vi "TCP-IP Link._Test_Node2.vi"() -> ()   [LabVIEW 2024, in "EQMF.lvlib" / "TCP-IP.lvlib"]
uses:
  TCP-IP.lvlib
  Controls/TCP-IP Link.Config.ctl
  Controls/TCP-IP Link.Status.ctl
  Queues/Q.Element.ctl
  Controls/TCP-IP Link.Options.ctl
  Controls/TCP-IP Link.Packet Format.ctl
  Queues/Queue Utils.lvlib
panel:
  in  "Options":T1={"Status Notify En"=TRUE, "Auto Connect"=TRUE, "Packet Format"=enum."First 2 Bytes is Length (U16)"}
  in  "Clear Error":bool
  in  "Name":string="Node2"
  out "Error Out":errorcluster
  out "Status Active":bool
  in  "Get Status":bool
  in  "Set Config":bool
  in  "Disconnect":bool
  in  "Connect":bool
  in  "Status":T3={"Cmd"="Task", "Sub"="TCP-IP Status", "Data1"=variant, "Data2"=variant}
  in  "Rcv Data":T3={"Cmd"="Task", "Sub"="TCP-IP Rcv", "Data1"=variant, "Data2"=variant}
  out "Status":T4
  in  "Config":T5={"IP"="127.0.0.1", "Port"=8510, "Listener"=FALSE}
  out "Connected":bool
  in  "Exit":bool
  out "Rcv Data":string
  in  "Send Data":string
  in  "Send":bool
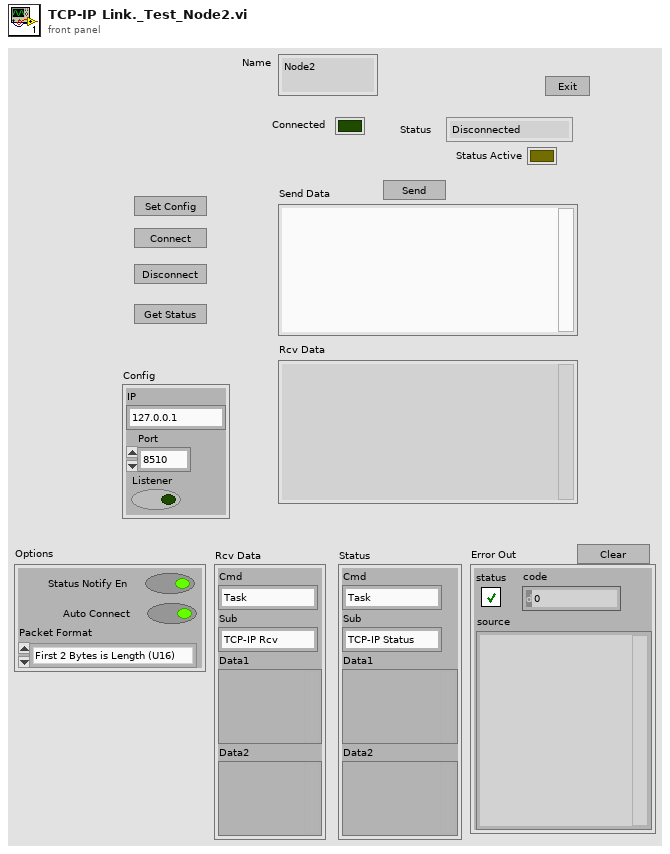
[diagram p1: front panel]
types:
  T1 = typedef "EQMF.lvlib/TCP-IP.lvlib/TCP-IP Link.Options.ctl" = cluster{"Status Notify En":bool, "Auto Connect":bool, "Packet Format":T2}
  T2 = typedef "EQMF.lvlib/TCP-IP.lvlib/TCP-IP Link.Packet Format.ctl" = enum16{"First 2 Bytes is Length (U16)", "First 3 Chars is Length"}
  T3 = typedef "EQMF.lvlib/Queue Utils.lvlib/Q.Element.ctl" = cluster{"Cmd":string, "Sub":string, "Data1":variant, "Data2":variant}
  T4 = typedef "EQMF.lvlib/TCP-IP.lvlib/TCP-IP Link.Status.ctl" = enum16{"Disconnected", "Connected", "Connecting", "Failed to Connect", "Listening"}
  T5 = typedef "EQMF.lvlib/TCP-IP.lvlib/TCP-IP Link.Config.ctl" = cluster{"IP":string, "Port":u16, "Listener":bool}
  T6 = enum8{"Enabled", "Disabled", "Disabled and Grayed Out"}
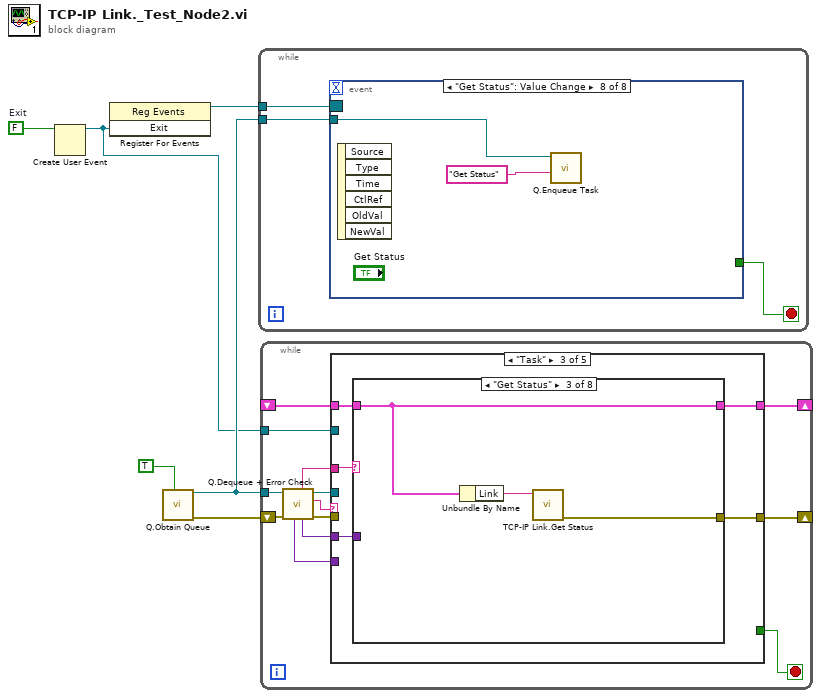
[diagram p0: block diagram]
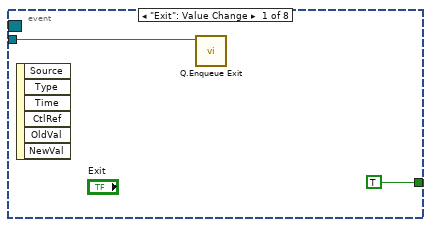
[diagram p2: hidden frame]
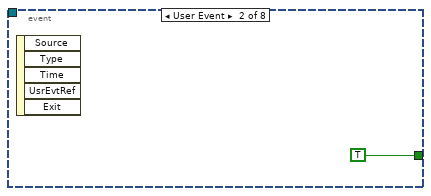
[diagram p3: hidden frame]
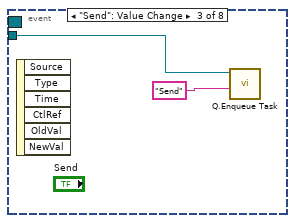
[diagram p4: hidden frame]
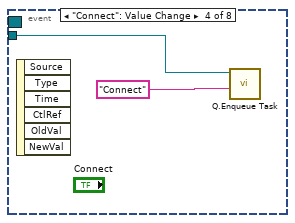
[diagram p5: hidden frame]
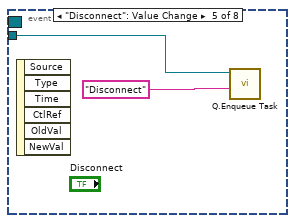
[diagram p6: hidden frame]
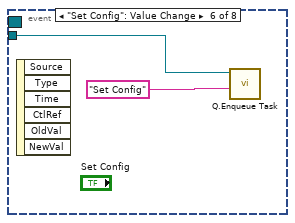
[diagram p7: hidden frame]
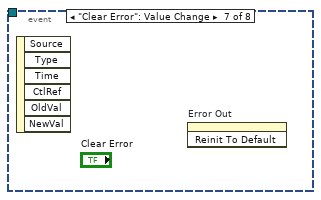
[diagram p8: hidden frame]
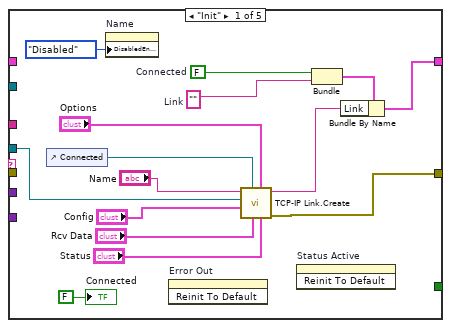
[diagram p9: hidden frame]
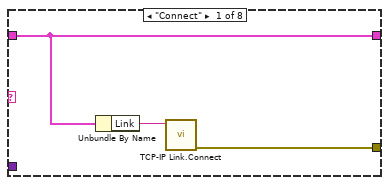
[diagram p11: hidden frame]
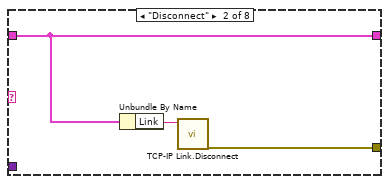
[diagram p12: hidden frame]
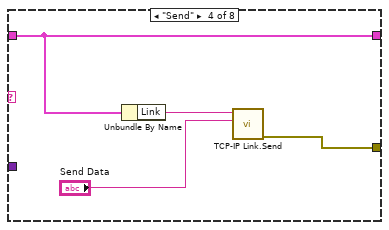
[diagram p13: hidden frame]
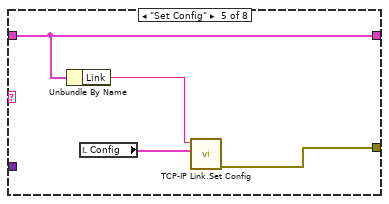
[diagram p14: hidden frame]
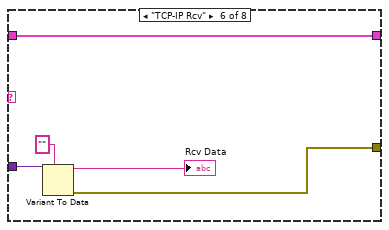
[diagram p15: hidden frame]
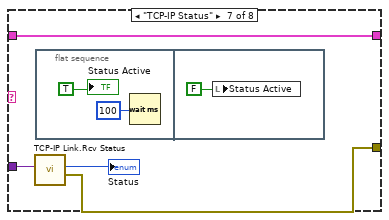
[diagram p16: hidden frame]
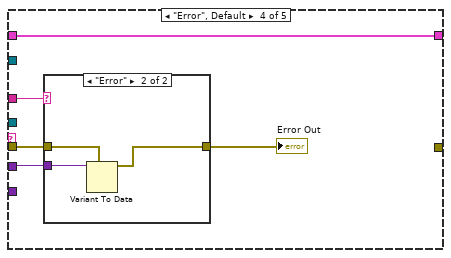
[diagram p18: hidden frame]
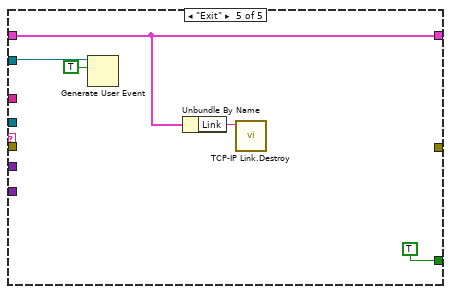
[diagram p20: hidden frame]
diagram:
  w3 = FALSE  # Exit
  n1 = Create User Event(user event datatype=w3) -> (user event=w2:refnum<user-event>)  [unwired: 1 in, 1 out]
  n2 = register-events(w2) -> (reference out=w4:refnum<event-registration>)  [unwired: 2 in, 1 out]
  n3 = call "Q.Obtain Queue.vi"("Enqueue Init"=TRUE) -> ("error out"=w1:errorcluster, "Q Out"=w6:refnum<queue>)  [unwired: 8 in, 1 out]
  n4 = while {
    tunnel: w6 -> [w9]
    tunnel: w4 -> [w7]
    stop <- w8 stop-if-true
    n5 = event shown="[7] \"Get Status\": Value Change" {
      selector: w7 -> [_ _ _ _ _ _ _ _]
      dyn-events: _ -> [_ _ _ _ _ _ _ _]
      timeout: _ -> [_ _ _ _ _ _ _ _]
      tunnel: w9 -> [w11 _ w14 w16 w18 w20 _ w22]
      tunnel: [TRUE TRUE _ _ _ _ _ _] -> w8
      event "Exit": Value Change {
        n6 = event-data() -> ()  [unwired: 1 in, 6 out]
        n7 = call "Q.Enqueue Exit.vi"("Q In"=w11) -> ()  [unwired: 9 in, 2 out]
      }
      event User Event {
        n8 = event-data() -> ()  [unwired: 1 in, 5 out]
      }
      event "Send": Value Change {
        n9 = event-data() -> ()  [unwired: 1 in, 6 out]
        n10 = call "Q.Enqueue Task.vi"("Task Name"="Send", "Q In"=w14) -> ()  [unwired: 8 in, 2 out]
      }
      event "Connect": Value Change {
        n11 = event-data() -> ()  [unwired: 1 in, 6 out]
        n12 = call "Q.Enqueue Task.vi"("Task Name"="Connect", "Q In"=w16) -> ()  [unwired: 8 in, 2 out]
      }
      event "Disconnect": Value Change {
        n13 = event-data() -> ()  [unwired: 1 in, 6 out]
        n14 = call "Q.Enqueue Task.vi"("Task Name"="Disconnect", "Q In"=w18) -> ()  [unwired: 8 in, 2 out]
      }
      event "Set Config": Value Change {
        n15 = event-data() -> ()  [unwired: 1 in, 6 out]
        n16 = call "Q.Enqueue Task.vi"("Task Name"="Set Config", "Q In"=w20) -> ()  [unwired: 8 in, 2 out]
      }
      event "Clear Error": Value Change {
        n17 = event-data() -> ()  [unwired: 1 in, 6 out]
        n18 = invoke on="Error Out" class="Clust (strict)" method="Reinit To Default"() -> ()  [unwired: 3 in, 3 out]
      }
      event "Get Status": Value Change {
        n19 = event-data() -> ()  [unwired: 1 in, 6 out]
        n20 = call "Q.Enqueue Task.vi"("Task Name"="Get Status", "Q In"=w22) -> ()  [unwired: 8 in, 2 out]
      }
    }
  }
  n21 = while {
    tunnel: w6 -> [w34]
    shift-right: [w27] -> _
    shift-left: _ -> [w28]
    tunnel: w2 -> [w26]
    shift-right: [w23] -> _
    shift-left: w1 -> [w25]
    stop <- w29 stop-if-true
    n22 = call "Q.Dequeue + Error Check.vi"("Error In"=w25, "Q In"=w34) -> ("error out"=w24:errorcluster, "Cmd"=w35:string, "Q Out"=w33:refnum<queue>, "Data1"=w31:variant, "Sub"=w32:string, "Data2"=w30:variant)  [unwired: 4 in]
    n23 = case shown="\"Task\"" w35 {
      tunnel: w33 -> [w43 _ _ _ _]
      tunnel: w32 -> [_ _ w56 w90 _]
      tunnel: w31 -> [_ _ w55 w89 _]
      tunnel: w30 -> [_ _ _ _ _]
      tunnel: [_ _ _ _ TRUE] -> w29
      tunnel: w28 -> [_ w51 w54 w91 w96]
      tunnel: [w46 w51 w53 w91 w96] -> w27
      tunnel: w26 -> [_ _ _ _ w99]
      tunnel: w24 -> [_ _ _ w88 _]
      tunnel: [w39 _ w52 _ _] -> w23
      frame "Init" {
        w48 = ""  # Link
        w49 = FALSE  # Connected
        n24 = control-ref of="Connected"() -> (w45:refnum<vi>)
        n25 = property on="Name" class="Str"("DisabledEnum"=T6."Disabled" ("Disabled")) -> ()  [unwired: 2 in, 2 out]
        n26 = invoke on="Error Out" class="Clust (strict)" method="Reinit To Default"() -> ()  [unwired: 3 in, 3 out]
        n27 = call "TCP-IP Link.Create.vi"("Status Element"="Status", "Options"="Options", "Rcv Data Element"="Rcv Data", "StatusCtrlRef"=w45, "Config"="Config", "Q_RcvData"=w43, "Control Q Name"="Name") -> ("Error Out"=w39:errorcluster, "Control Q Name Dup"=w44:string)  [unwired: 3 in]
        n28 = invoke on="Status Active" class="Bool (strict)" method="Reinit To Default"() -> ()  [unwired: 3 in, 3 out]
        n29 = Bundle("Connected"=w49, "Link"=w48) -> (w47:cluster{"Connected":bool, "Link":string})  [unwired: 1 in]
        n30 = Bundle By Name(cluster=w47, "Link"=w44) -> (w46:cluster{"Connected":bool, "Link":string})
        "Connected" <- FALSE ("Connected")
      }
      frame "Reset" {
      }
      frame "Task" {
        n31 = case shown="\"Get Status\"" w56 {
          tunnel: w55 -> [_ _ _ _ _ w78 w81 _]
          tunnel: w54 -> [w59 w62 w65 w69 w73 w75 w82 w86]
          tunnel: [w59 w62 w65 w69 w73 w75 w82 w86] -> w53
          tunnel: [w57 w60 w63 w66 w70 w74 w79 _] -> w52
          frame "Connect" {
            n32 = Unbundle By Name(w59) -> ("Link"=w58:string)
            n33 = call "TCP-IP Link.Connect.vi"("Link Q Name"=w58) -> ("error out"=w57:errorcluster)  [unwired: 10 in]
          }
          frame "Disconnect" {
            n34 = Unbundle By Name(w62) -> ("Link"=w61:string)
            n35 = call "TCP-IP Link.Disconnect.vi"("Link Q Name"=w61) -> ("error out"=w60:errorcluster)  [unwired: 10 in]
          }
          frame "Get Status" {
            n36 = Unbundle By Name(w65) -> ("Link"=w64:string)
            n37 = call "TCP-IP Link.Get Status.vi"("Link Q Name"=w64) -> ("error out"=w63:errorcluster)  [unwired: 10 in]
          }
          frame "Send" {
            n38 = Unbundle By Name(w69) -> ("Link"=w68:string)
            n39 = call "TCP-IP Link.Send.vi"("Data"="Send Data", "Link Q Name"=w68) -> ("error out"=w66:errorcluster)  [unwired: 9 in]
          }
          frame "Set Config" {
            n40 = Unbundle By Name(w73) -> ("Link"=w72:string)
            n41 = local read "Config"() -> (w71:T5)
            n42 = call "TCP-IP Link.Set Config.vi"("TCP-IP Config"=w71, "Link Q Name"=w72) -> ("error out"=w70:errorcluster)  [unwired: 9 in]
          }
          frame "TCP-IP Rcv" {
            n43 = Variant To Data(type="", Variant=w78) -> (data=→"Rcv Data":string, error out=w74:errorcluster)  [unwired: 1 in]
          }
          frame "TCP-IP Status" {
            n44 = call "TCP-IP Link.Rcv Status.vi"("Data"=w81) -> ("error out"=w79:errorcluster, "Status"=→"Status":T4)  [unwired: 9 in]
            n45 = flat-sequence {
              frame #0 {
                n46 = Wait (ms)(milliseconds to wait=u32 100) -> ()  [unwired: 1 out]
                "Status Active" <- TRUE
              }
              frame #1 {
                n47 = local write "Status Active"(FALSE ("Status Active")) -> ()
              }
            }
          }
          frame Default {
          }
        }
      }
      frame "Error", Default {
        n48 = case shown="\"Error\"" w90 {
          tunnel: w89 -> [_ w95]
          tunnel: w88 -> [w92 w94]
          tunnel: [w92 w93] -> w87
          frame Default {
          }
          frame "Error" {
            n49 = Variant To Data(type=w94, Variant=w95) -> (data=w93:errorcluster)  [unwired: 1 in, 1 out]
          }
        }
        "Error Out" <- w87
      }
      frame "Exit" {
        n50 = Generate User Event(user event=w99, event data cluster=TRUE ("event data")) -> ()  [unwired: 2 in, 2 out]
        n51 = Unbundle By Name(w96) -> ("Link"=w97:string)
        n52 = call "TCP-IP Link.Destroy.vi"("Q Name"=w97) -> ()  [unwired: 10 in, 1 out]
      }
    }
  }
